vi "Get Object Metadata.vi"(8 "error in (no error)":errorcluster, 10 "Object Key":string, 11 "Bucket in":refnum<class "Bucket.lvclass">) -> (0 "error out":errorcluster, 2 "Data":string, 3 "Bucket out":refnum<class "Bucket.lvclass">)   [LabVIEW 2015]
uses:
  Bucket.lvclass
  Core/HTTP Request/Request Options.ctl
  Core/HTTP Request/Name Value Pair.ctl
  Core/HTTP Request/Region handling.ctl
  Core/HTTP Request/URL formatting.ctl
  Bucket.lvclass/Bucket.ctl
  Read Name.vi
  Core/HTTP Request/HTTP Request.lvclass
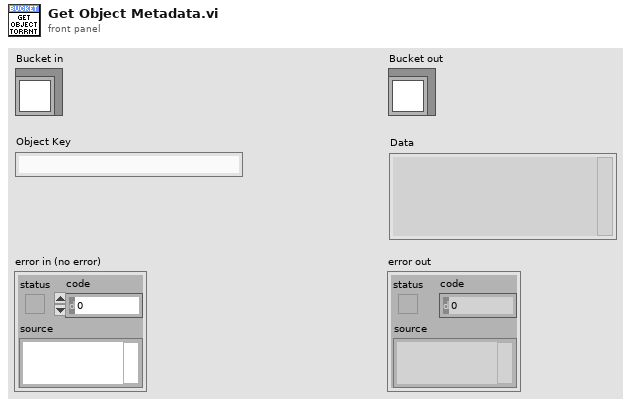
[diagram p1: front panel]
types:
  T1 = typedef "NI_AWS_Core.lvlib/HTTP Request.lvclass/Name Value Pair.ctl" = cluster{"name":string, "value":string}
  T2 = typedef "NI_AWS_Core.lvlib/HTTP Request.lvclass/Region handling.ctl" = enum16{"use region everywhere", "use region (authentication only)", "use region (URL only)", "ignore region everwhere"}
  T3 = typedef "NI_AWS_Core.lvlib/HTTP Request.lvclass/Request Options.ctl" = cluster{"request headers":T1[], "request parameters":T1[], "request body":string, "region handling":T2, "URL formatting":T4}
  T4 = typedef "NI_AWS_Core.lvlib/HTTP Request.lvclass/URL formatting.ctl" = enum16{"region-", "region."}
  T5 = typedef "NI_AWS_Core.lvlib/HTTP Request.lvclass/Response.ctl" = cluster{"Headers":string, "Body":string}
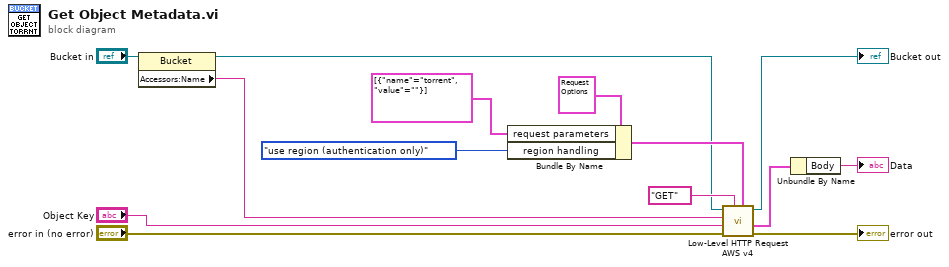
[diagram p0: block diagram]
diagram:
  n1 = property class="Bucket"(reference="Bucket in") -> (reference out=w2:refnum<class "Bucket.lvclass">, "Accessors:Name"=w13:string)  [unwired: 1 in, 1 out]
  n2 = Bundle By Name(cluster=T3 {"request headers"=[], "request parameters"=[], "request body"="", "region handling"=enum."use region everywhere", "URL formatting"=enum."region."} ("Request Options"), "request parameters"=T1[] [{"name"="torrent", "value"=""}], "region handling"=Region_handling."use region (authentication only)") -> (w4:T3)
  n3 = call "Low-Level HTTP Request AWS v4.vi"("Request Options"=w4, "HTTP-Verb"="GET", "error in (no error)"="error in (no error)", "URL Suffix"="Object Key", "URL Prefix"=w13, "AWS Core in"=w2) -> ("error out"=→"error out":errorcluster, "Response"=w6:T5, "AWS Core out"=→"Bucket out":refnum<class "Bucket.lvclass">)  [unwired: 2 in, 1 out]
  n4 = Unbundle By Name(w6) -> ("Body"=→"Data":string)
